vi "Read 1D Array.vi"(8 "error in (no error)":errorcluster, 11 "Data1D in":refnum<class "Data1D.lvclass">) -> (0 "error out":errorcluster, 2 "1D Array":dbl[](array[numeric]), 3 "Data1D out":refnum<class "Data1D.lvclass">)   [LabVIEW 2014, in "Data1D.lvclass"]
uses:
  Data1D.lvclass
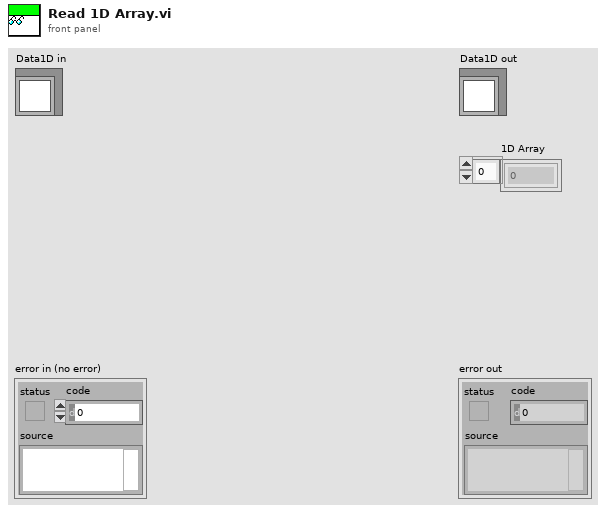
[diagram p1: front panel]
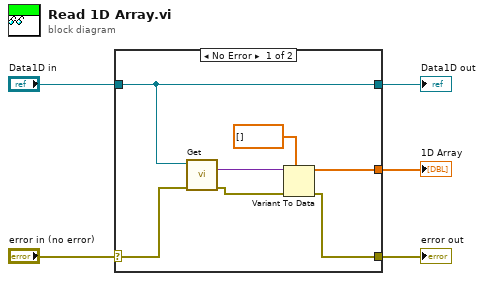
[diagram p0: block diagram]
diagram:
  n1 = case shown="No Error" "error in (no error)" {
    selector: "error in (no error)" -> [w9 w13]
    tunnel: [w8 w13] -> w4
    tunnel: [w12 w14] -> w2
    tunnel: "Data1D in" -> [w12 w14]
    tunnel: [w6 _] -> w1
    frame No Error {
      n2 = call-dynamic "Get.vi"("error in (no error)"=w9, "AbstractData in"=w12) -> ("error out"=w10:errorcluster, "Data"=w11:variant)  [unwired: 7 in, 1 out]
      n3 = Variant To Data(error in=w10, type=dbl[] [] ("1D Array 2"), Variant=w11) -> (data=w6:dbl[], error out=w8:errorcluster)
    }
    frame Error {
    }
  }
  "error out" <- w4
  "Data1D out" <- w2
  "1D Array" <- w1
